vi "Header String Constant.vi"() -> (1 "Multiple Header String":string, 3 "Single Header String":string)   [LabVIEW 2020, in "Multi Error Cluster.lvlib"]
doc: "Return the values for the single and multi-error header."
uses:
  <vilib>/MultiError/TokenizeJSON/Multi Error Cluster.lvlib
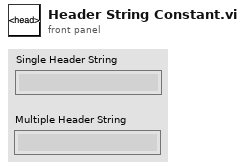
[diagram p1: front panel]
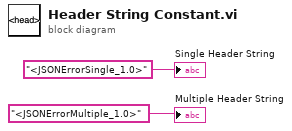
[diagram p0: block diagram]
diagram:
  "Single Header String" <- "<JSONErrorSingle_1.0>" ("source")
  "Multiple Header String" <- "<JSONErrorMultiple_1.0>" ("source")
